vi "ort_fit_calcSlopeDissipation.vi"() -> (3 "debugOut":T1)   [LabVIEW 2016]
uses:
  <vilib>/rvi/Emulation/niFpgaEmulationIsFPGAContextNoSignature.vi
  <vilib>/rvi/Emulation/niFpgaSctlEmulationGetInTimedLoop.vi
  <vilib>/rvi/errors/niFpgaSetErrorForExecOnDevCompSimple.vi
  <vilib>/rvi/eio/common/nirviEmuReportErrorAndStop.vi
  <vilib>/rvi/DataTransferAndStorage/Container/Common/niFpgaContainerGetUniqueNameForEmu.vi
  <vilib>/rvi/FIFO/Fifo_Resource/nirvififoEmulationSetSize.vi
  <vilib>/rvi/FIFO/Fifo_Resource/nirviFifoEmulationQueueMgr.vi
  <instcachedir>/0/nirviFifoEmulationQueueMgr_E5CAEC123FF24DC58D834DCA3CDAA9B5.lvgen/nirviFifoEmulationQueueMgr_E5CAEC123FF24DC58D834DCA3CDAA9B5_008.vi
  <vilib>/rvi/FIFO/Fifo_Resource/nirvififoEmulationDetermineInputValidOut.vi
  <vilib>/rvi/FIFO/Fifo_Resource/nirvififoEmulationCreateLock.vi
  <vilib>/rvi/Emulation/niFpgaProcessEmulError.vi
  <vilib>/rvi/FIFO/Fifo_Resource/nirvififoEmulationObtainLock.vi
  <vilib>/rvi/FIFO/Fifo_Resource/nirvififoEmulationReleaseLock.vi
  <vilib>/rvi/occurrence/nirviWaitOnOccurrenceBase.vi
  <vilib>/rvi/errors/nirviReportUnexpectedCaseInternalError.vi
  <vilib>/rvi/errors/nirviReportUnexpectedCaseInternalError (U32).vi
  <instcachedir>/0/nirviFifoEmulationQueueMgr_E5CAEC123FF24DC58D834DCA3CDAA9B5.lvgen/nirviFifoEmulationQueueMgr_E5CAEC123FF24DC58D834DCA3CDAA9B5_001.vi
  <vilib>/Utility/error.llb/Clear Errors.vi
  <instcachedir>/0/nirviFifoEmulationQueueMgr_E5CAEC123FF24DC58D834DCA3CDAA9B5.lvgen/nirviFifoEmulationQueueMgr_E5CAEC123FF24DC58D834DCA3CDAA9B5_002.vi
  <instcachedir>/0/nirviFifoEmulationQueueMgr_E5CAEC123FF24DC58D834DCA3CDAA9B5.lvgen/nirviFifoEmulationQueueMgr_E5CAEC123FF24DC58D834DCA3CDAA9B5_006.vi
  <vilib>/rvi/FXPMathLib/FxpInterpret/XNode/nifxpmath_Interpret.xnode
  <vilib>/rvi/DataTransferAndStorage/Container/XNode/niFpgaContainer.xnode
  <vilib>/rvi/FIFO/Fifo_Resource/nirvififoEmulationWrite.vi
  <vilib>/rvi/FIFO/Fifo_Resource/nirvififoEmulationRead.vi
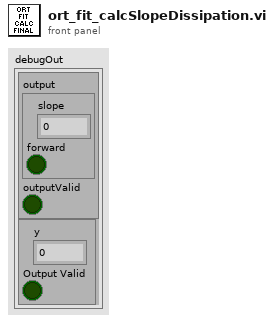
[diagram p1: front panel]
types:
  T1 = cluster{cluster{"output":cluster{"slope":fxp<+/-,22,1>, "forward":bool}, "outputValid":bool}, cluster{"y":fxp<+/-,32,1>, "Output Valid":bool}}
  T2 = cluster{"linSum":i32, "wtSum":fxp<+/-,54,34>, "count":u16, "forward":bool}
  T3 = cluster{"output":cluster{"slope":fxp<+/-,22,1>, "forward":bool}, "outputValid":bool}
  T4 = cluster{cluster{"output":cluster{"slope":fxp<+/-,22,1>, "forward":bool}, "outputValid":bool}, cluster{"y":fxp<+/-,32,10>, "Output Valid":bool}}
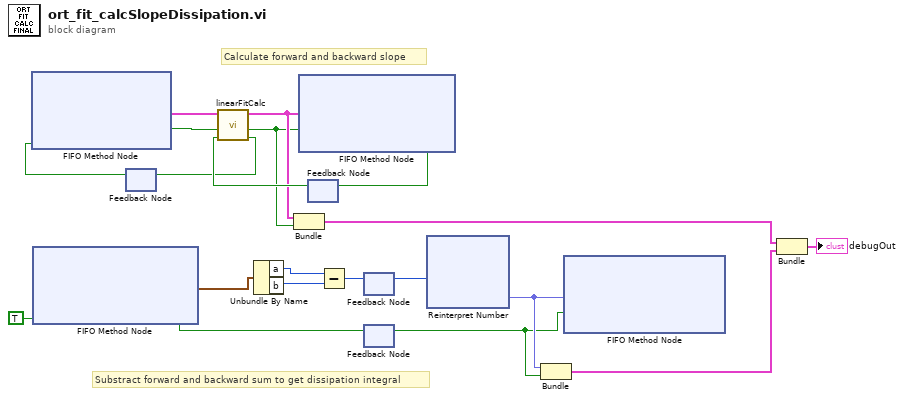
[diagram p0: block diagram]
diagram:
  # "Calculate forward and backward slope"
  # "Substract forward and backward sum to get dissipation integral"
  n1 = xnode ("FIFO Method Node")("Ready for Output"=TRUE) -> ("Element"=w17:cluster{"a":i32, "b":i32}, "Output Valid"=w19:bool)  [unwired: 1 in, 1 out]
  n2 = feedback #1() -> (w11:bool)  [unwired: 1 in]
  n3 = xnode ("FIFO Method Node")("Ready for Output"=w11) -> ("Element"=w8:T2, "Output Valid"=w9:bool)  [unwired: 1 in, 1 out]
  n4 = Unbundle By Name(w17) -> ("a"=w16:i32, "b"=w15:i32)
  n5 = feedback #2() -> (w13:bool)  [unwired: 1 in]
  n6 = call "linearFitCalc.vi"("ready for output (T)"=w13, "inputValid"=w9, "input"=w8) -> ("ready for input"=w10:bool, "outputValid"=w4:bool, "output"=w5:cluster{"slope":fxp<+/-,22,1>, "forward":bool})  [unwired: 6 in]
  n7 = feedback-in #1(w10) -> ()
  n8 = Bundle("output"=w5, "outputValid"=w4) -> (w3:T3)  [unwired: 1 in]
  n9 = xnode ("FIFO Method Node")("Element"=w5, "Input Valid"=w4) -> ("Ready for Input"=w12:bool)  [unwired: 1 in, 1 out]
  n10 = feedback-in #2(w12) -> ()
  n11 = Subtract(x=w16, y=w15) -> (x-y=w14:i32)
  n12 = feedback #3() -> (w18:i32)  [unwired: 1 in]
  n13 = feedback-in #3(w14) -> ()
  n14 = feedback #4() -> (w6:bool)  [unwired: 1 in]
  n15 = feedback-in #4(w19) -> ()
  n16 = xnode "Reinterpret Number"("x"=w18) -> ("y"=w7:fxp<+/-,32,10>)
  n17 = Bundle("y"=w7, "Output Valid"=w6) -> (w2:cluster{"y":fxp<+/-,32,10>, "Output Valid":bool})  [unwired: 1 in]
  n18 = xnode ("FIFO Method Node")("Element"=w7, "Input Valid"=w6) -> ()  [unwired: 1 in, 2 out]
  n19 = Bundle(w3, w2) -> (→"debugOut":T4)  [unwired: 1 in]
